vi "U3 PWM16 Loop.vi"(8 "error in":errorcluster, 9 "PWM Duty Cycle [%]":dbl=50.0 format="%.4f") -> (0 "error out":errorcluster)   [LabVIEW 2021]
panel:
  in  "stop":bool
  out "aTimerValues":u16[](array[numeric])
  in  "FirstFound":bool=TRUE
  in  "Address":string="1"
  out "Error Message":string
  # "Demonstrates 1 timer channel of 16-bit PWM output on FIO4 with a frequency of 40.7 Hz. \nUpdates the duty cycle every 500 ms in a loop."
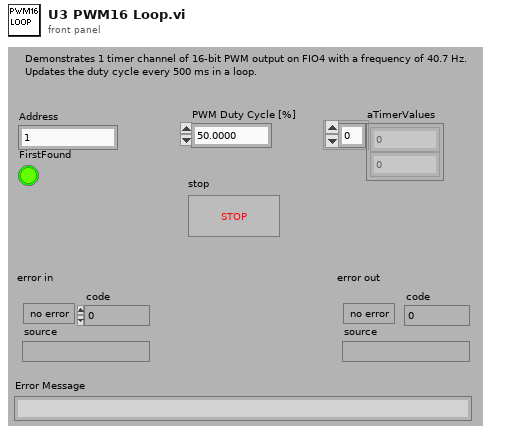
[diagram p1: front panel]
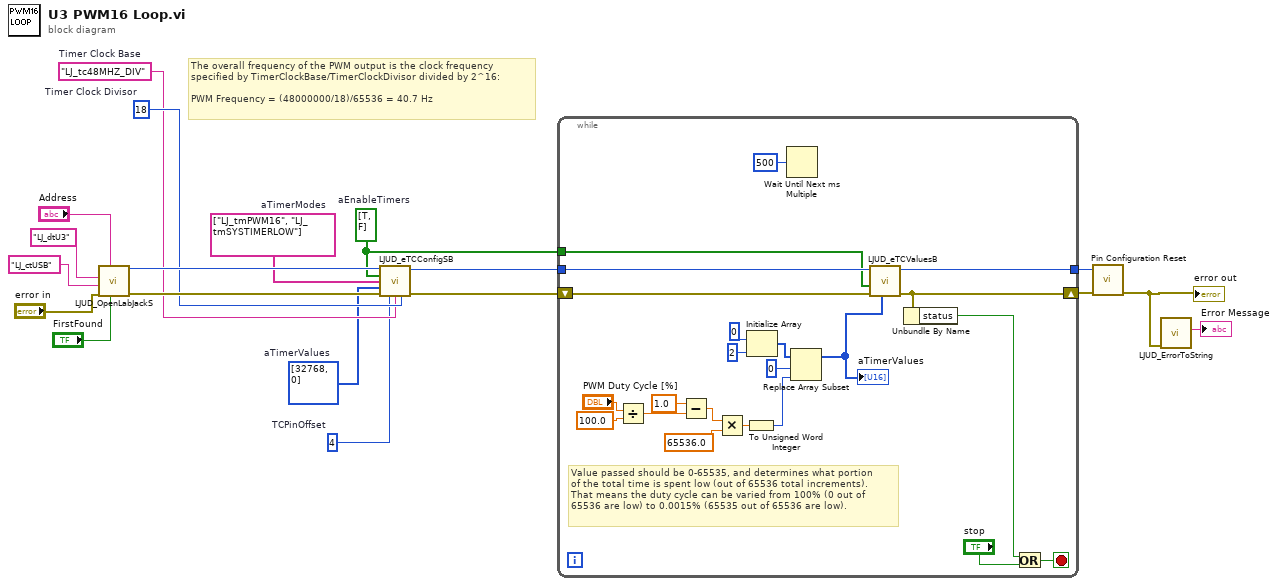
[diagram p0: block diagram]
diagram:
  w4 = u16[] [32768, 0]  # aTimerValues
  w8 = 4  # TCPinOffset
  w5 = bool[] [TRUE, FALSE]  # aEnableTimers
  w10 = 18  # Timer Clock Divisor
  w9 = "LJ_tc48MHZ_DIV"  # Timer Clock Base
  w11 = string[] ["LJ_tmPWM16", "LJ_tmSYSTIMERLOW"]  # aTimerModes
  # "The overall frequency of the PWM output is the clock frequency\nspecified by TimerClockBase/TimerClockDivisor divided by 2^16:\n\nPWM Frequency = (48000000/18)/65536 = 40.7 Hz"
  n1 = call "LJUD_OpenLabJackS.vi"("FirstFound"="FirstFound", "Address"="Address", "error in"="error in", "ConnectionType"="LJ_ctUSB", "DeviceType"="LJ_dtU3") -> ("error out"=w13:errorcluster, "Handle"=w12:i32)  [unwired: 4 in, 1 out]
  n2 = call "LJUD_eTCConfigSB.vi"("Handle In"=w12, "aEnableTimers"=w5, "aTimerModes"=w11, "aTimerValues"=w4, "error in"=w13, "TCPinOffset"=w8, "TimerClockBase"=w9, "TimerClockDivisor"=w10) -> ("Handle Out"=w6:i32, "error out"=w7:errorcluster)  [unwired: 6 in]
  n3 = while {
    shift-right: [w23] -> w3
    shift-left: w7 -> [w39]
    tunnel: w6 -> [w41]
    tunnel: w5 -> [w40]
    tunnel: [w20] -> w1
    stop <- w24 stop-if-true
    # "Value passed should be 0-65535, and determines what portion\nof the total time is spent low (out of 65536 total increments).\nThat means the duty cycle can be varied from 100% (0 out of\n65536 are low) to 0.0015% (65535 out of 65536 are low)."
    n4 = Divide(x="PWM Duty Cycle [%]", y=100.0) -> (x/y=w30:dbl)
    n5 = Subtract(x=1.0, y=w30) -> (x-y=w32:dbl)
    n6 = Multiply(x=w32, y=65536.0) -> (x*y=w37:dbl)
    n7 = To Unsigned Word Integer(number=w37) -> (unsigned 16bit integer=w38:u16)
    n8 = Initialize Array(u16 0 ("PWM Timer Value"), 2 ("Dimension Size")) -> (w35:u16[])
    n9 = Wait Until Next ms Multiple(millisecond multiple=u32 500) -> ()  [unwired: 1 out]
    n10 = Replace Array Subset(array=w35, new element=w38, index=0 ("Index")) -> (w25:u16[])
    "aTimerValues" <- w25
    n11 = call "LJUD_eTCValuesB.vi"("aTimerValues Write"=w25, "error in"=w39, "aUpdateResetTimers"=w40, "Handle In"=w41) -> ("error out"=w23:errorcluster, "Handle Out"=w20:i32)  [unwired: 4 in, 2 out]
    n12 = Unbundle By Name(w23) -> ("status"=w22:bool)
    n13 = Or(x=w22, y="stop") -> (x .or. y?=w24:bool)
  }
  n14 = call "Pin Configuration Reset.vi"("error in"=w3, "Handle In"=w1) -> ("error out"=w2:errorcluster)  [unwired: 8 in, 1 out]
  "error out" <- w2
  n15 = call "LJUD_ErrorToString.vi"("error in"=w2) -> ("String"=→"Error Message":string)  [unwired: 10 in]
